vi "Reply.vi"(7 "Sender":refnum<class "Sender.lvclass">, 9 "Is Priority":bool, 10 "Msg":refnum<class "Msg.lvclass">, 11 "TEMPLATE Actor in":refnum<class "TEMPLATE Actor.lvclass">) -> (0 "Error out":errorcluster)   [LabVIEW 2025, in "TEMPLATE Actor.lvlib" / "TEMPLATE Actor.lvclass"]
uses:
  TEMPLATE Actor.lvclass
  <vilib>/Nathan Davis/jettl/jettl/jettl/Sender/Sender/Sender.lvclass
  <vilib>/Nathan Davis/jettl/jettl/jettl/Msg/Msg.lvclass
  TEMPLATE Actor.lvclass/TEMPLATE Actor.ctl
  <vilib>/Nathan Davis/jettl/jettl/jettl/Actor/Actor/Actor.lvclass
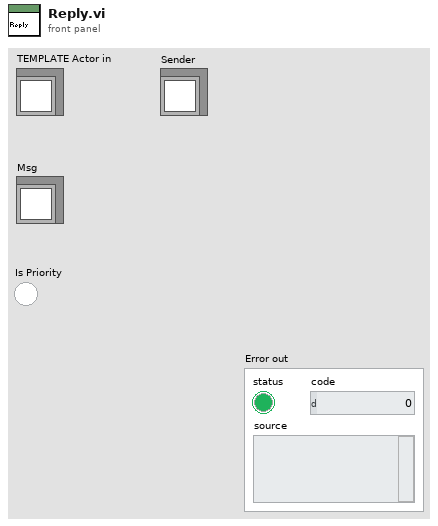
[diagram p1: front panel]
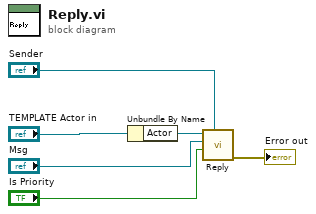
[diagram p0: block diagram]
diagram:
  n1 = Unbundle By Name("TEMPLATE Actor in") -> ("Actor"=w1:refnum<class "Actor.lvclass">)
  n2 = call-dynamic "Reply.vi"("Sender"="Sender", "Is Priority"="Is Priority", "Msg"="Msg", "Actor in"=w1) -> ("Error out"=→"Error out":errorcluster)  [unwired: 7 in]
